vi "destroy.vi"(8 "error in (no error)":errorcluster, 11 "ClientBuilder in":refnum<class "ClientBuilder.lvclass">) -> (0 "error out":errorcluster)   [LabVIEW 2020, in "reqwest.lvlib" / "ClientBuilder.lvclass"]
uses:
  ClientBuilder.lvclass
  ClientBuilder.lvclass/ClientBuilder.ctl
  lv_reqwest_64.so
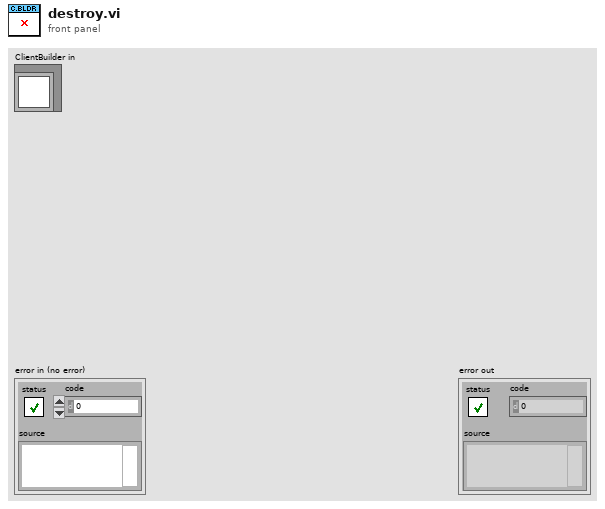
[diagram p1: front panel]
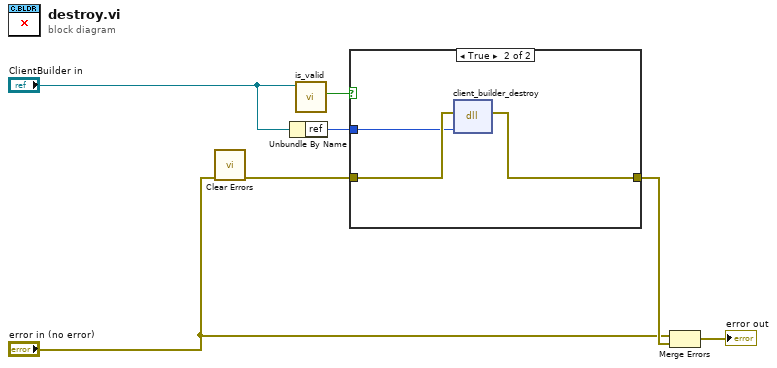
[diagram p0: block diagram]
diagram:
  n1 = call <vilib>:"Clear Errors.vi"("error in (no error)"="error in (no error)") -> ("error out"=w6:errorcluster)  [unwired: 5 in, 1 out]
  n2 = Unbundle By Name("ClientBuilder in") -> ("ref"=w3:u64)
  n3 = call "is_valid.vi"("Client in"="ClientBuilder in") -> ("valid-ref?"=w1:bool)  [unwired: 10 in]
  n4 = case shown="True" w1 {
    tunnel: [w8 w11] -> w7
    tunnel: w6 -> [w8 w10]
    tunnel: w3 -> [_ w9]
    frame False {
    }
    frame True {
      n5 = dll-call lib="home/jim-kring/Projects/reqwest-rs-labview/lv_src/lv_reqwest_*.*" fn="client_builder_destroy"(error in=w10, "ptr"=w9) -> (error out=w11:errorcluster)  [unwired: 4 in, 1 out]
    }
  }
  n6 = Merge Errors("error in (no error)", w7) -> (→"error out":errorcluster)
